vi "BuildNewProjectPath.vi"(9 "File Prefix":string caption="文件前缀", 10 "Project Root":path caption="项目根目录", 11 "Project Name":string caption="项目名称") -> (1 "Error Message":string caption="错误信息", 2 "Valid?":bool caption="合法？", 3 "New Project Path":path caption="新项目路径")   [LabVIEW 2016]
uses:
  <vilib>/Utility/error.llb/whitespace.ctl
  <vilib>/Utility/Multibyte/NI_Multibyte Utilities.lvlib
panel:
  in  "Trailing Whitespace":string="“项目根目录”包含的文件夹名称尾部带有空白字符。" caption="尾部空白"
  in  "Bad Characters in Path Error Message":string="“项目根目录”中包含不可作为文件路径的非法字符。" caption="路径包含非法字符错误信息"
  in  "Non-empty Root Folder Error Message":string="指定的“项目根目录”非空。如新建一个项目，必须将路径设定为空目录。如设定的路径所指目录不存在，则LabVIEW将自动创建该目录。" caption="非空根目录错误信息"
  in  "Empty Project Name Error Message":string="“项目名称”为空。" caption="空项目名称错误信息"
  in  "Invalid Path Explanation":string="目标路径无效，无法复制。" caption="无效路径解释"
  in  "Blank Path Explanation":string="目标路径为空，无法复制。" caption="空路径解释"
  in  "Invalid Path Error Message":string="“项目根目录”无效。" caption="无效路径错误信息"
  in  "Bad Prefix Error Message":string="“文件名前缀”中包含不可作为文件名的非法字符。" caption="非法前缀错误信息"
  in  "Bad Filename Error Message":string="“项目名称”中包含不可作为文件名的非法字符。" caption="非法文件名错误信息"
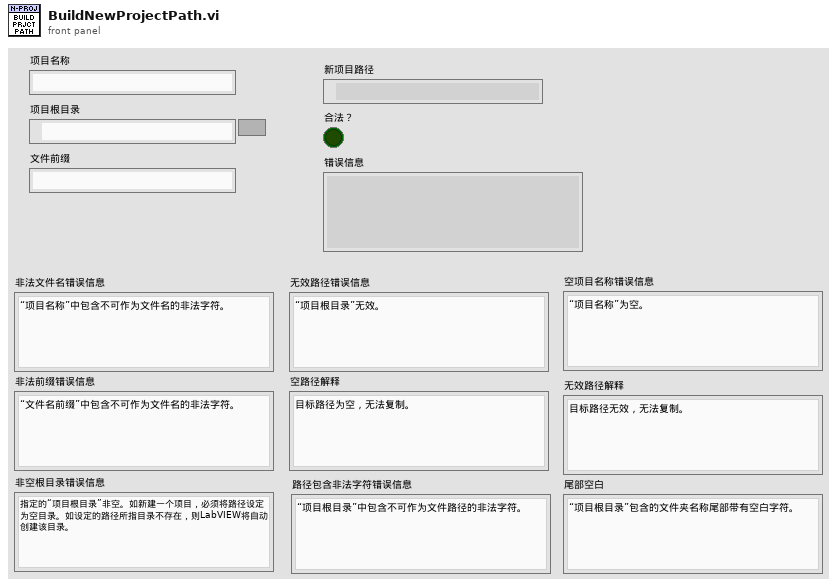
[diagram p1: front panel]
types:
  T1 = typedef "whitespace.ctl" = u16
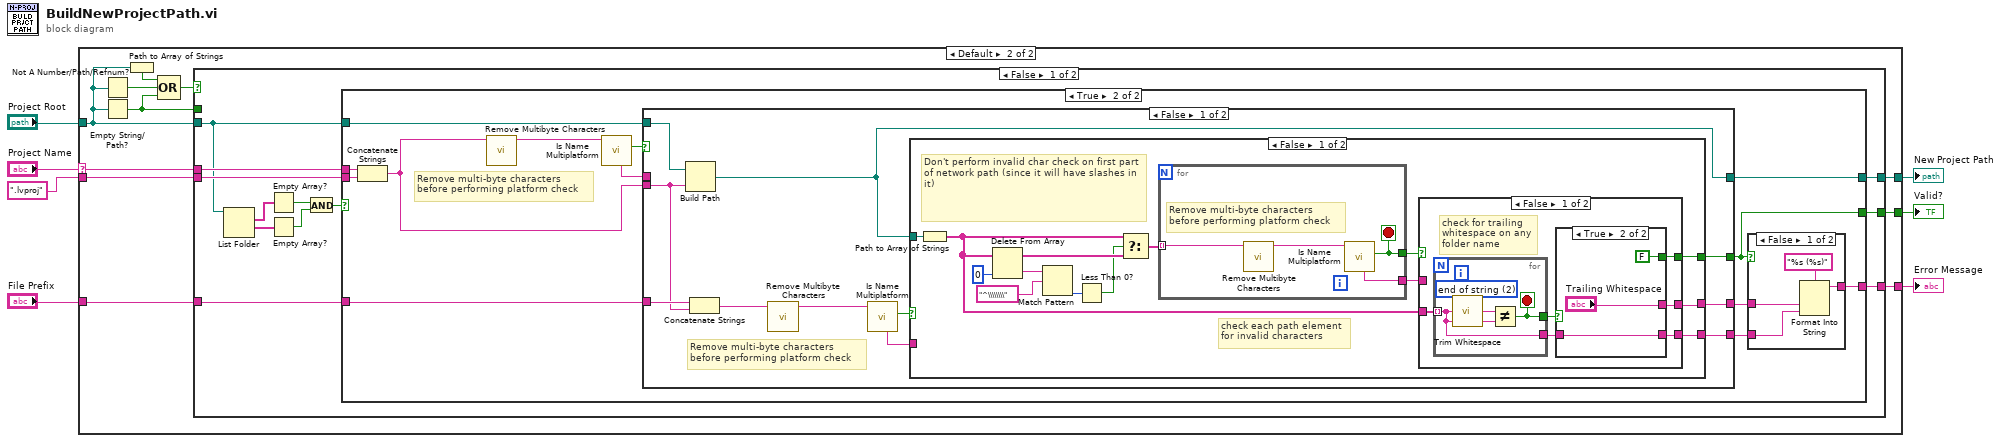
[diagram p0: block diagram]
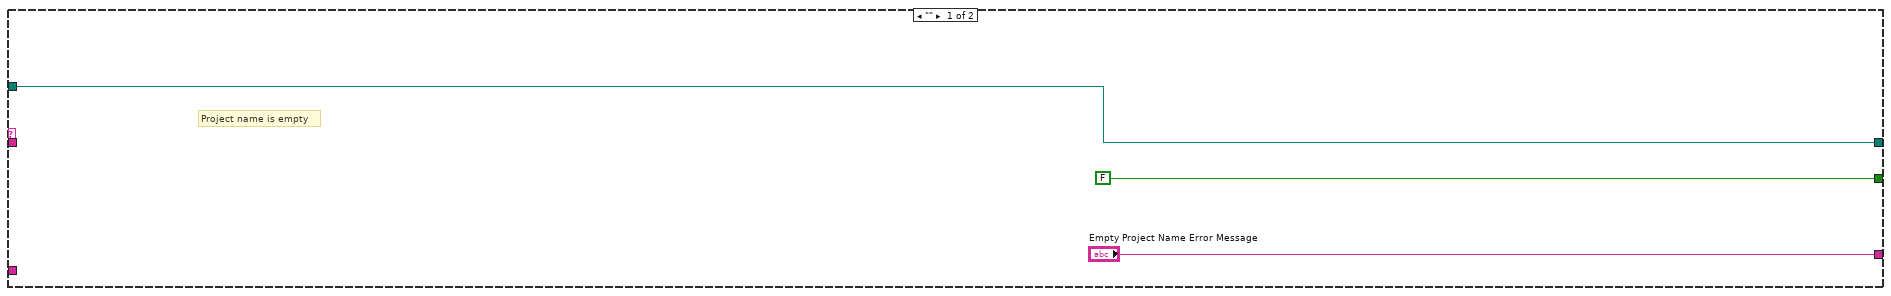
[diagram p2: hidden frame]
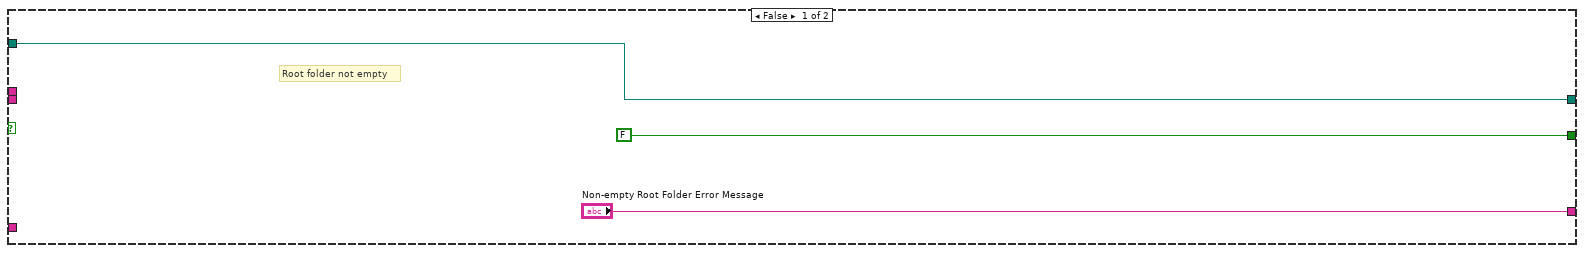
[diagram p3: hidden frame]
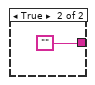
[diagram p4: hidden frame]
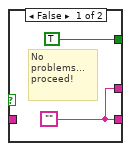
[diagram p5: hidden frame]
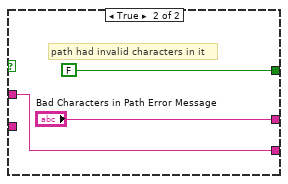
[diagram p6: hidden frame]
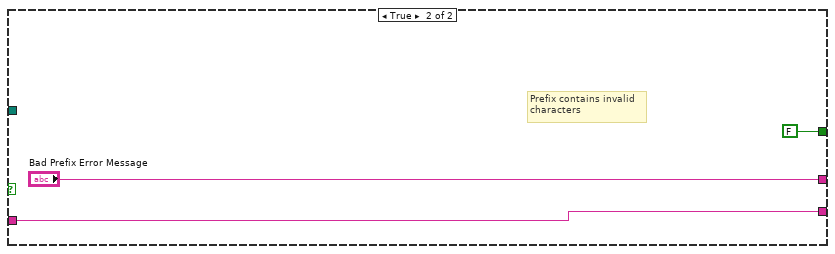
[diagram p7: hidden frame]
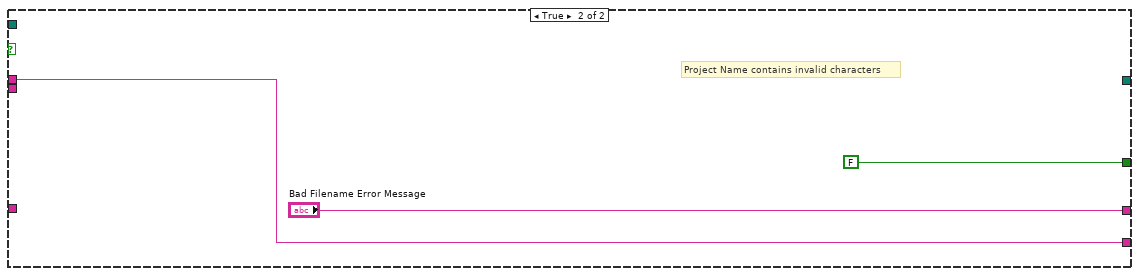
[diagram p8: hidden frame]
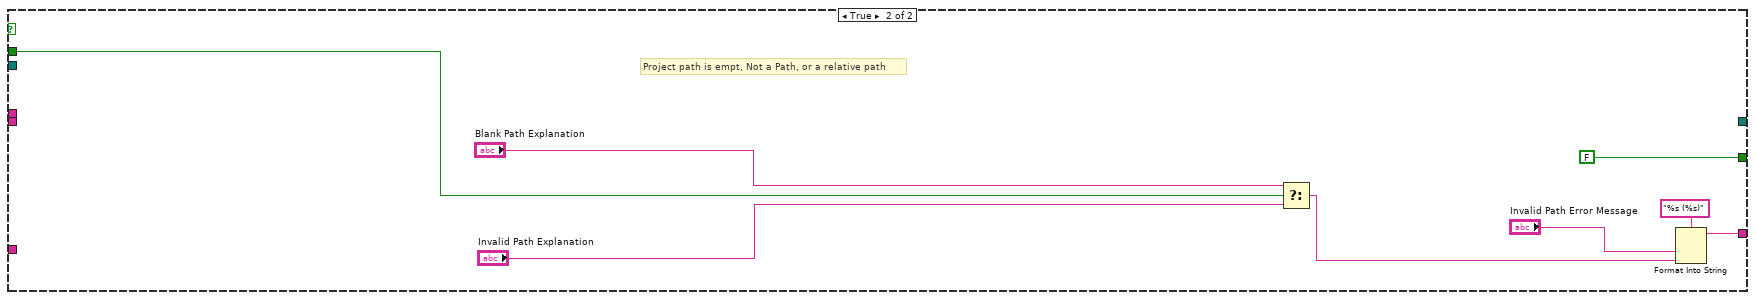
[diagram p9: hidden frame]
diagram:
  n1 = case shown="Default" "Project Name" {
    selector: "Project Name" -> [_ w16]
    tunnel: ["Empty Project Name Error Message" w15] -> w7
    tunnel: ".lvproj" ("string") -> [_ w21]
    tunnel: [w10 w20] -> w5
    tunnel: [FALSE ("Valid?") w19] -> w4
    tunnel: "File Prefix" -> [_ w18]
    tunnel: "Project Root" -> [w10 w14]
    frame "" {
      # "Project name is empty"
    }
    frame Default {
      n2 = Not A Number/Path/Refnum?(number/path/refnum=w14) -> (NaN/Path/Refnum?=w12:bool)
      n3 = Empty String/Path?(string/path=w14) -> (empty?=w11:bool)
      n4 = Path to Array of Strings(0:w14) -> (1:w13:bool)  [unwired: 1 out]
      n5 = Compound Arithmetic op=OR(w13, w12, w11) -> (w17:bool)
      n6 = case shown="False" w17 {
        tunnel: w16 -> [w33 _]
        tunnel: w21 -> [w32 _]
        tunnel: [w31 _] -> w20
        tunnel: [w24 FALSE] -> w19
        tunnel: w14 -> [w29 _]
        tunnel: w18 -> [w30 _]
        tunnel: [w23 w111] -> w15
        tunnel: w11 -> [_ w110]
        frame False {
          n7 = List Folder(path=w29) -> (filenames=w28:string[], folder names=w27:string[])  [unwired: 3 in, 2 out]
          n8 = Empty Array?(array=w28) -> (empty?=w26:bool)
          n9 = Empty Array?(array=w27) -> (empty?=w25:bool)
          n10 = And(x=w26, y=w25) -> (x .and. y?=w22:bool)
          n11 = case shown="True" w22 {
            tunnel: w33 -> [_ w49]
            tunnel: w32 -> [_ w46]
            tunnel: [w36 w45] -> w31
            tunnel: w30 -> [_ w44]
            tunnel: w29 -> [w36 w43]
            tunnel: [FALSE ("Valid?") w40] -> w24
            tunnel: ["Non-empty Root Folder Error Message" w39] -> w23
            frame False {
              # "Root folder not empty"
            }
            frame True {
              # "Remove multi-byte characters\nbefore performing platform check"
              n12 = Concatenate Strings(w49, w46) -> (w38:string)
              n13 = call <vilib>:"Remove Multibyte Characters.vi"("String"=w38) -> ("String with Multibyte Removed"=w37:string)  [unwired: 8 in, 2 out]
              n14 = call <vilib>:"Is Name Multiplatform.vi"("filename"=w37) -> ("filename had conflict"=w48:bool, "problem description"=w47:string)  [unwired: 6 in, 3 out]
              n15 = case shown="False" w48 {
                tunnel: [w65 "Bad Filename Error Message"] -> w42
                tunnel: w47 -> [_ w107]
                tunnel: [w61 w107] -> w41
                tunnel: [w64 FALSE ("Valid?")] -> w40
                tunnel: w38 -> [w58 _]
                tunnel: [w57 _] -> w45
                tunnel: w43 -> [w60 _]
                tunnel: w44 -> [w59 _]
                frame False {
                  # "Remove multi-byte characters\nbefore performing platform check"
                  n16 = Build Path(base path=w60, name or relative path=w58) -> (appended path=w57:path)
                  n17 = Concatenate Strings(w59, w58) -> (w55:string)
                  n18 = call <vilib>:"Remove Multibyte Characters.vi"("String"=w55) -> ("String with Multibyte Removed"=w56:string)  [unwired: 8 in, 2 out]
                  n19 = call <vilib>:"Is Name Multiplatform.vi"("filename"=w56) -> ("filename had conflict"=w63:bool, "problem description"=w62:string)  [unwired: 6 in, 3 out]
                  n20 = case shown="False" w63 {
                    tunnel: [w78 "Bad Prefix Error Message"] -> w65
                    tunnel: [w79 FALSE] -> w64
                    tunnel: w62 -> [_ w103]
                    tunnel: [w77 w103] -> w61
                    tunnel: w57 -> [w76 _]
                    frame False {
                      # "Don't perform invalid char check on first part of network path (since it will have slashes in it)"
                      # "check each path element\nfor invalid characters"
                      n21 = Path to Array of Strings(0:w76) -> (2:w69:string[])  [unwired: 1 out]
                      n22 = Delete From Array(array=w69, index=0) -> (deleted portion=w72:string, array with subset deleted=w67:string[])  [unwired: 1 in]
                      n23 = Match Pattern(string=w72, regular expression="^\\\\\\\\") -> (offset past match=w70:i32)  [unwired: 1 in, 3 out]
                      n24 = Less Than 0?(x=w70) -> (x < 0?=w66:bool)
                      n25 = Select(t=w69, s=w66, f=w67) -> (s? t:f=w68:string[])
                      n26 = for {
                        tunnel: w68 -> [w99] mode=indexing
                        tunnel: [w101] -> w74
                        tunnel: [w100] -> w75
                        stop <- w100 stop-if-true
                        # "Remove multi-byte characters\nbefore performing platform check"
                        n27 = call <vilib>:"Remove Multibyte Characters.vi"("String"=w99) -> ("String with Multibyte Removed"=w98:string)  [unwired: 8 in, 2 out]
                        n28 = call <vilib>:"Is Name Multiplatform.vi"("filename"=w98) -> ("filename had conflict"=w100:bool, "problem description"=w101:string)  [unwired: 6 in, 3 out]
                      }
                      n29 = case shown="False" w75 {
                        tunnel: [w85 FALSE] -> w79
                        tunnel: [w84 "Bad Characters in Path Error Message"] -> w78
                        tunnel: [w82 w96] -> w77
                        tunnel: w74 -> [_ w96]
                        tunnel: w69 -> [w83 _]
                        frame False {
                          # "check for trailing whitespace on any folder name"
                          n30 = for {
                            tunnel: w83 -> [w91] mode=indexing
                            tunnel: [w92] -> w81
                            tunnel: [w91] -> w80
                            stop <- w92 stop-if-true
                            w94 = T1 2 items=["both", "start of string", "end of string"] ("location (both)")
                            n31 = call <vilib>:"Trim Whitespace.vi"("string"=w91, "location (both)"=w94) -> ("trimmed string"=w93:string)
                            n32 = Not Equal?(x=w93, y=w91) -> (x != y?=w92:bool)
                          }
                          n33 = case shown="True" w81 {
                            tunnel: [TRUE FALSE] -> w85
                            tunnel: [w86 "Trailing Whitespace"] -> w84
                            tunnel: [w86 w89] -> w82
                            tunnel: w80 -> [_ w89]
                            frame False {
                              w86 = ""
                              # "No problems... proceed!"
                            }
                            frame True {
                            }
                          }
                        }
                        frame True {
                          # "path had invalid characters in it"
                        }
                      }
                    }
                    frame True {
                      # "Prefix contains invalid\ncharacters"
                    }
                  }
                }
                frame True {
                  # "Project Name contains invalid characters"
                }
              }
              n34 = case shown="False" w40 {
                tunnel: [w53 ""] -> w39
                tunnel: w42 -> [w51 _]
                tunnel: w41 -> [w50 _]
                frame False {
                  n35 = Format Into String(format string="%s (%s)" ("string"), w51, w50) -> (resulting string=w53:string)  [unwired: 2 in, 1 out]
                }
                frame True {
                }
              }
            }
          }
        }
        frame True {
          # "Project path is empt, Not a Path, or a relative path"
          n36 = Select(t="Blank Path Explanation", s=w110, f="Invalid Path Explanation") -> (s? t:f=w112:string)
          n37 = Format Into String(format string="%s (%s)" ("string"), "Invalid Path Error Message", w112) -> (resulting string=w111:string)  [unwired: 2 in, 1 out]
        }
      }
    }
  }
  "Valid?" <- w4
  "Error Message" <- w7
  "New Project Path" <- w5
